vi "Write SetPoint.vi"(4 "Setpoint":dbl format="%_4g", 6 "Previous Setpoint":dbl=nan format="%_4g", 7 "Unit ID (A)":string="A", 8 "error in":errorcluster, 9 "Software Version":u8, 10 "Controller Info out":T1={"Controller Full Scale"=nan, "Controller Select"=0, "Control Range"=enum."Normal"} {"Controller Select" items=["No controller"=0, "Volumetric Flow"=36, "Mass Flow"=37, "Absolute Pressure"=34, "Gauge Pressure"=38, "Differential Pressure"=39]}, 11 "VISA Session In":refnum<visa-resource-name>="Alicat") -> (0 "error out":errorcluster, 1 "Data frame returned":string, 2 "Controller Info out":T1={"Controller Full Scale"=nan, "Controller Select"=0, "Control Range"=enum."Normal"} {"Controller Select" items=["No controller"=0, "Volumetric Flow"=36, "Mass Flow"=37, "Absolute Pressure"=34, "Gauge Pressure"=38, "Differential Pressure"=39]}, 3 "VISA Session Out":refnum<visa-resource-name>)   [LabVIEW 2015]
doc: "Writes a new setpoint to the specified Alicat device. If device type and/or fullscale range is unspecified, the device is queried. If device is not a controller, or setpoint is NaN, setpoint update is skipped.\n\nIt also performs a check to see if the setpoint is different from previously written value. If not, the setpoint command is skipped. The previous setpint should be obtained by use of a shift register.\n\nThis VI also returns the data frame after a write command is sent, which can then be parsed using the \"Parse Data Frame\" VI. If the write is skipped, the data frame return will be an empty string constant instead."
uses:
  <vilib>/Instr/_visa.llb/VISA Flush IO Buffer Mask.ctl
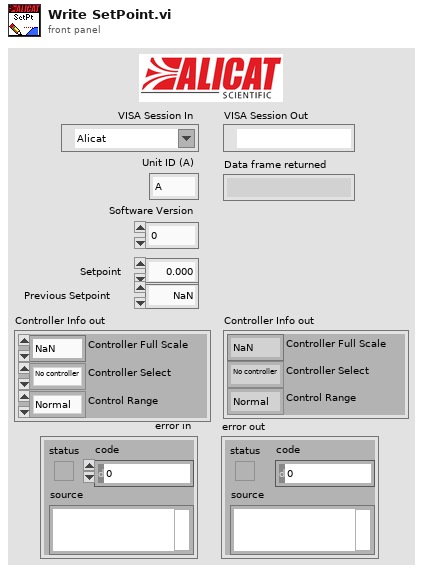
[diagram p1: front panel]
types:
  T1 = cluster{"Controller Full Scale":dbl, "Controller Select":u16, "Control Range":enum16{"Normal", "Inverted", "Bidirectional", "Unknown"}}
  T2 = enum16{"Normal", "Inverted", "Bidirectional", "Unknown"}
  T3 = typedef "VISA Flush IO Buffer Mask.ctl" = u16
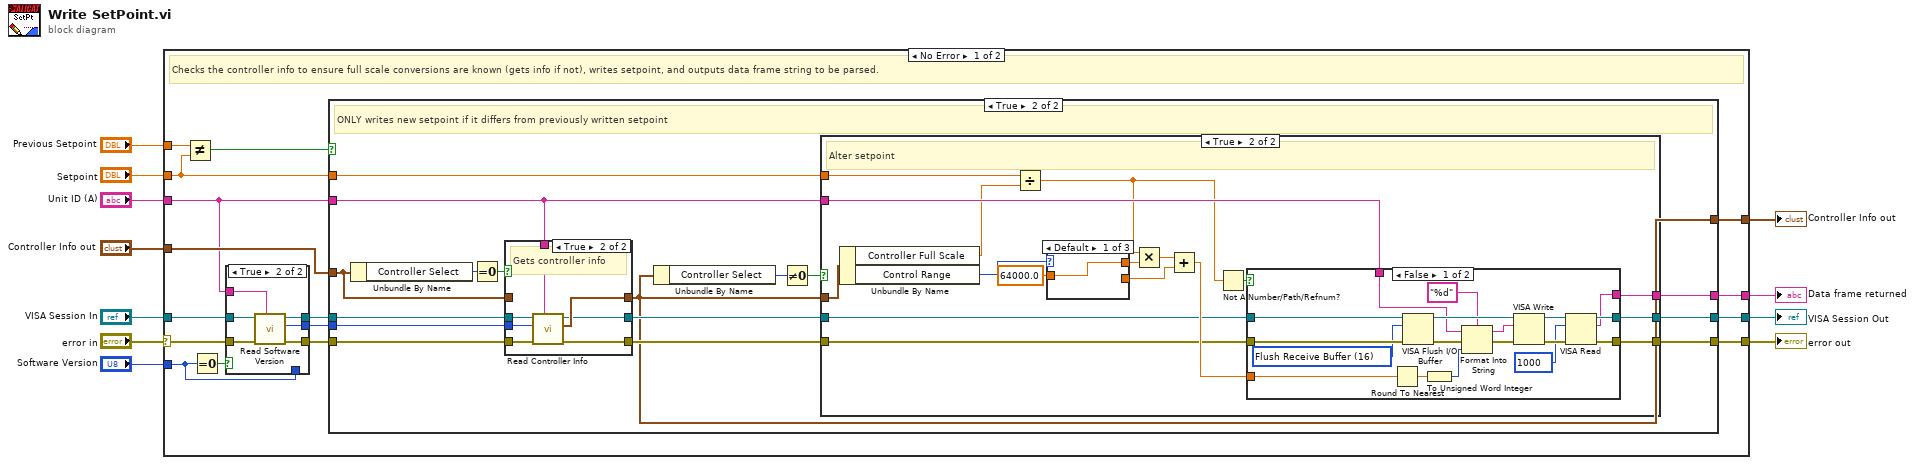
[diagram p0: block diagram]
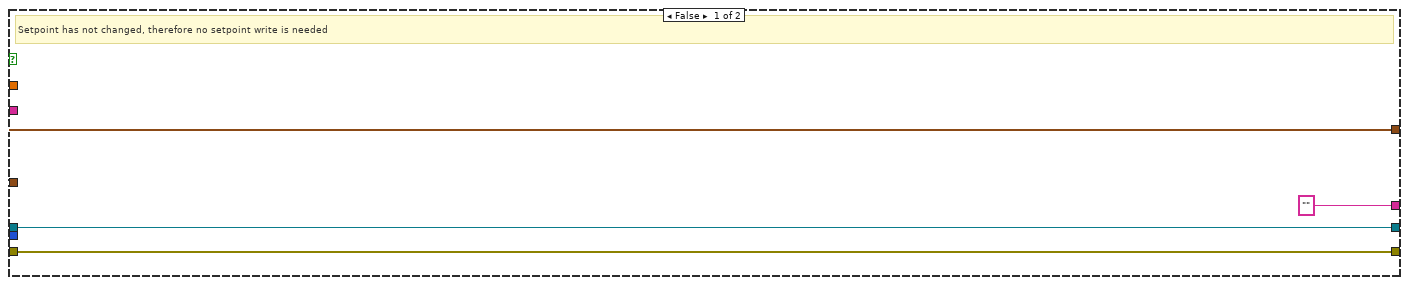
[diagram p3: hidden frame]
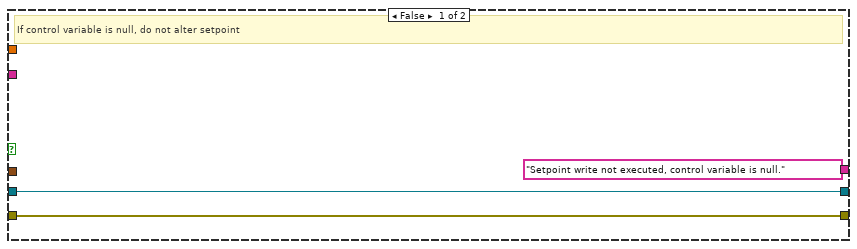
[diagram p4: hidden frame]
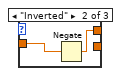
[diagram p5: hidden frame]
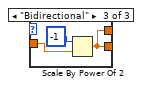
[diagram p6: hidden frame]
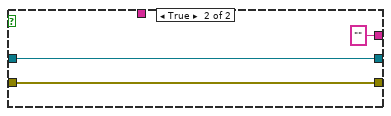
[diagram p7: hidden frame]
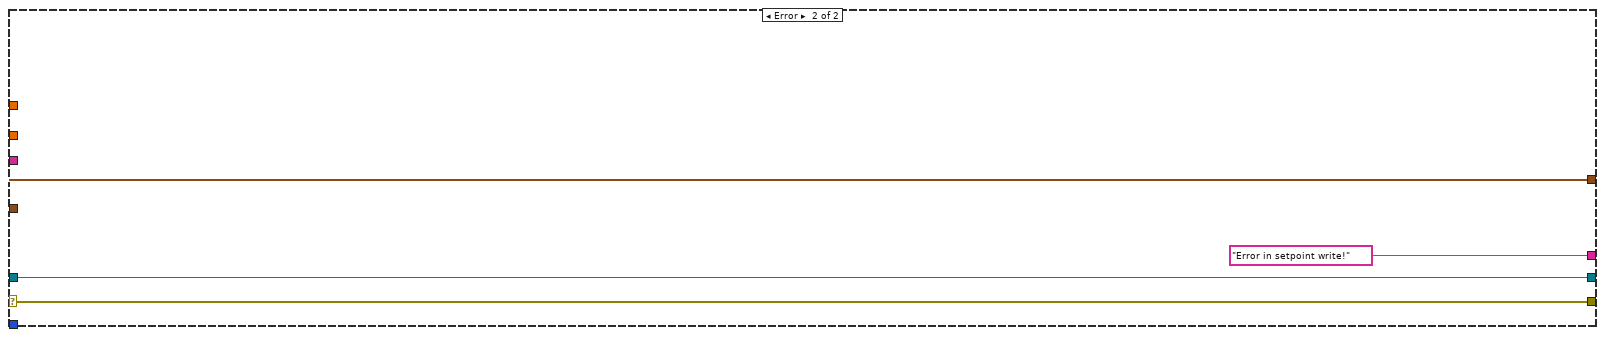
[diagram p9: hidden frame]
diagram:
  n1 = case shown="No Error" "error in" {
    selector: "error in" -> [w17 w114]
    tunnel: [w27 w115] -> w11
    tunnel: [w26 w114] -> w10
    tunnel: [w25 "Error in setpoint write!" ("read buffer")] -> w9
    tunnel: "Controller Info out" -> [w24 w117]
    tunnel: "VISA Session In" -> [w18 w115]
    tunnel: "Setpoint" -> [w21 _]
    tunnel: [w23 w117] -> w2
    tunnel: "Unit ID (A)" -> [w16 _]
    tunnel: "Previous Setpoint" -> [w22 _]
    tunnel: "Software Version" -> [w15 _]
    frame No Error {
      # "Checks the controller info to ensure full scale conversions are known (gets info if not), writes setpoint, and outputs data frame string to be parsed."
      n2 = Not Equal?(x=w22, y=w21) -> (x != y?=w20:bool)
      n3 = Equal To 0?(x=w15) -> (x = 0?=w19:bool)
      n4 = case shown="True" w19 {
        tunnel: w17 -> [w29 w36]
        tunnel: w18 -> [w28 w35]
        tunnel: w16 -> [_ w34]
        tunnel: [w29 w33] -> w12
        tunnel: [w28 w32] -> w13
        tunnel: [w30 w31] -> w14
        tunnel: w15 -> [w30 _]
        frame False {
        }
        frame True {
          n5 = call "Read Software Version.vi"("Unit ID (A)"=w34, "error in"=w36, "VISA Session In"=w35) -> ("error out"=w33:errorcluster, "Software Version"=w31:u8, "VISA Session Out"=w32:refnum<visa-resource-name>)  [unwired: 6 in]
        }
      }
      n6 = case shown="True" w20 {
        tunnel: [w38 w56] -> w27
        tunnel: [w37 w55] -> w26
        tunnel: ["" ("read buffer") w54] -> w25
        tunnel: w24 -> [w40 w52]
        tunnel: w13 -> [w38 w51]
        tunnel: w21 -> [_ w50]
        tunnel: [w40 w43] -> w23
        tunnel: w16 -> [_ w49]
        tunnel: w12 -> [w37 w46]
        tunnel: w14 -> [_ w44]
        frame False {
          # "Setpoint has not changed, therefore no setpoint write is needed"
        }
        frame True {
          # "ONLY writes new setpoint if it differs from previously written setpoint"
          n7 = Unbundle By Name(w52) -> ("Controller Select"=w45:u16)
          n8 = Equal To 0?(x=w45) -> (x = 0?=w53:bool)
          n9 = case shown="True" w53 {
            tunnel: w52 -> [w106 _]
            tunnel: [w106 w113] -> w43
            tunnel: w49 -> [_ w112]
            tunnel: w51 -> [w105 w111]
            tunnel: w46 -> [w104 w110]
            tunnel: [w105 w109] -> w48
            tunnel: [w104 w108] -> w47
            tunnel: w44 -> [_ w107]
            frame False {
              # "Uses provided info"
            }
            frame True {
              # "Gets controller info"
              n10 = call "Read Controller Info.vi"("Unit ID (A)"=w112, "error in"=w110, "Software Version"=w107, "VISA Session In"=w111) -> ("error out"=w108:errorcluster, "Controller Info out"=w113:T1, "VISA Session Out"=w109:refnum<visa-resource-name>)  [unwired: 4 in, 1 out]
            }
          }
          n11 = Unbundle By Name(w43) -> ("Controller Select"=w41:u16)
          n12 = Not Equal To 0?(x=w41) -> (x != 0?=w42:bool)
          n13 = case shown="True" w42 {
            tunnel: [w58 w76] -> w56
            tunnel: [w57 w75] -> w55
            tunnel: ["Setpoint write not executed, control variable is null." ("read buffer") w72] -> w54
            tunnel: w50 -> [_ w71]
            tunnel: w43 -> [_ w70]
            tunnel: w49 -> [_ w69]
            tunnel: w48 -> [w58 w63]
            tunnel: w47 -> [w57 w62]
            frame False {
              # "If control variable is null, do not alter setpoint"
            }
            frame True {
              # "Alter setpoint"
              n14 = Unbundle By Name(w70) -> ("Controller Full Scale"=w61:dbl, "Control Range"=w60:T2)
              n15 = Divide(x=w71, y=w61) -> (x/y=w67:dbl)
              n16 = case shown="Default" w60 {
                tunnel: 64000.0 ("y") -> [w77 w79 w82]
                tunnel: [w77 w78 w80] -> w68
                tunnel: [_ _ w80] -> w65
                frame Default {
                }
                frame "Inverted" {
                  n17 = Negate(x=w79) -> (-x=w78:dbl)
                }
                frame "Bidirectional" {
                  n18 = Scale By Power Of 2(n=-1, x=w82) -> (x*2^n=w80:dbl)
                }
              }
              n19 = Multiply(x=w67, y=w68) -> (x*y=w66:dbl)
              n20 = Add(x=w66, y=w65) -> (x+y=w64:dbl)
              n21 = Not A Number/Path/Refnum?(number/path/refnum=w67) -> (NaN/Path/Refnum?=w74:bool)
              n22 = case shown="False" w74 {
                tunnel: [w97 w103] -> w76
                tunnel: [w92 w102] -> w75
                tunnel: w63 -> [w91 w103]
                tunnel: w62 -> [w90 w102]
                tunnel: w69 -> [w89 _]
                tunnel: w64 -> [w83 _]
                tunnel: [w84 "" ("read buffer")] -> w72
                frame False {
                  w85 = T3 16 items=["Flush Receive Buffer"=16, "Write Transmit Buffer to Device"=32, "Flush Receive Buffer (No I/O)"=64, "Flush Transmit Buffer"=128] ("Mask")
                  n23 = Round To Nearest(number=w83) -> (nearest integer value=w88:dbl)
                  n24 = VISA Flush I/O Buffer(VISA resource name=w91, mask (16)=w85, error in (no error)=w90) -> (VISA resource name out=w99:refnum<visa-resource-name>, error out=w94:errorcluster)
                  n25 = To Unsigned Word Integer(number=w88) -> (unsigned 16bit integer=w87:u16)
                  n26 = Format Into String(format string="%d", initial string=w89, error in=w94, w87) -> (resulting string=w95:string, error out=w93:errorcluster)
                  n27 = VISA Write(VISA resource name=w99, write buffer=w95, error in (no error)=w93) -> (VISA resource name out=w98:refnum<visa-resource-name>, error out=w100:errorcluster)  [unwired: 1 out]
                  n28 = VISA Read(VISA resource name=w98, byte count=u32 1000, error in (no error)=w100) -> (VISA resource name out=w97:refnum<visa-resource-name>, read buffer=w84:string, error out=w92:errorcluster)  [unwired: 1 out]
                }
                frame True {
                }
              }
            }
          }
        }
      }
    }
    frame Error {
    }
  }
  "error out" <- w10
  "VISA Session Out" <- w11
  "Data frame returned" <- w9
  "Controller Info out" <- w2
